vi "find lookahead point - Copy.vi"(6 "Lookahead Distance":dbl=4000.0, 11 "Path Data":T1={"Path"=[], "Target Velocities"=[], "Robot Location"=[], "Robot Angle (rad)"=0.0, "Curvature"=0.0, "Lookahead Point"=[3064.399009129367, 18229.833030071386], "Lookahead Index"=8.422809037111724, "Closest Point"=[], "Closest Point Index"=0, "Left Velocity"=0.0, "Right Velocity"=0.0, "Left Encoder Vel"=0, "Right Encoder Vel"=0, "Left Encoder Pos"=0, "Right Encoder Pos"=0}) -> (3 "Path Data":T1={"Path"=[], "Target Velocities"=[], "Robot Location"=[], "Robot Angle (rad)"=0.0, "Curvature"=0.0, "Lookahead Point"=[3064.399009129367, 18229.833030071386], "Lookahead Index"=8.422809037111724, "Closest Point"=[], "Closest Point Index"=0, "Left Velocity"=0.0, "Right Velocity"=0.0, "Left Encoder Vel"=0, "Right Encoder Vel"=0, "Left Encoder Pos"=0, "Right Encoder Pos"=0})   [LabVIEW 2018]
uses:
  path data.ctl
panel:
  out "a":dbl
  out "Lookahead Index":dbl=8.422809037111724
  out "Lookahead Point":dbl[](array[numeric])=[3064.399009129367, 18229.833030071386]
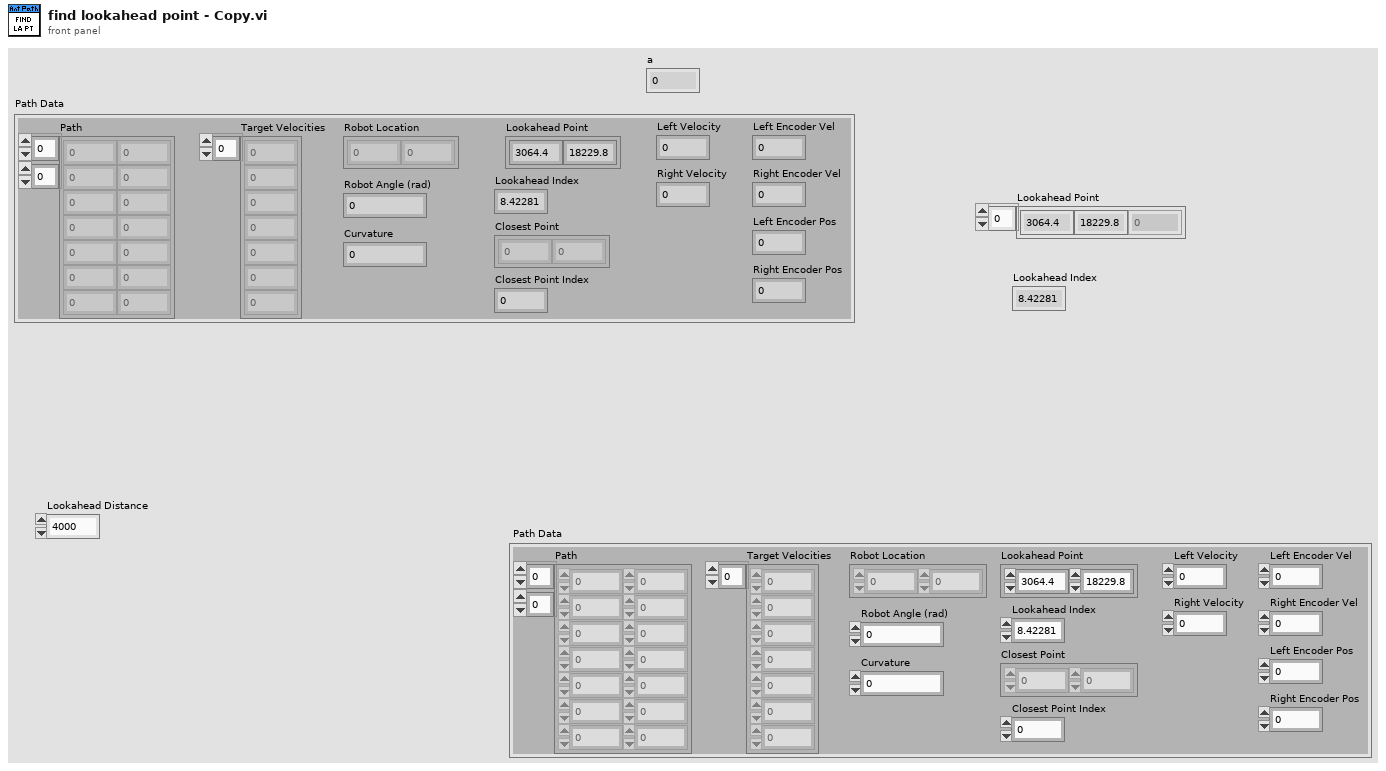
[diagram p1: front panel]
types:
  T1 = typedef "path data.ctl" = cluster{"Path":dbl[][], "Target Velocities":dbl[], "Robot Location":dbl[], "Robot Angle (rad)":dbl, "Curvature":dbl, "Lookahead Point":dbl[], "Lookahead Index":dbl, "Closest Point":dbl[], "Closest Point Index":i32, "Left Velocity":dbl, "Right Velocity":dbl, "Left Encoder Vel":i32, "Right Encoder Vel":i32, "Left Encoder Pos":i32, "Right Encoder Pos":i32}
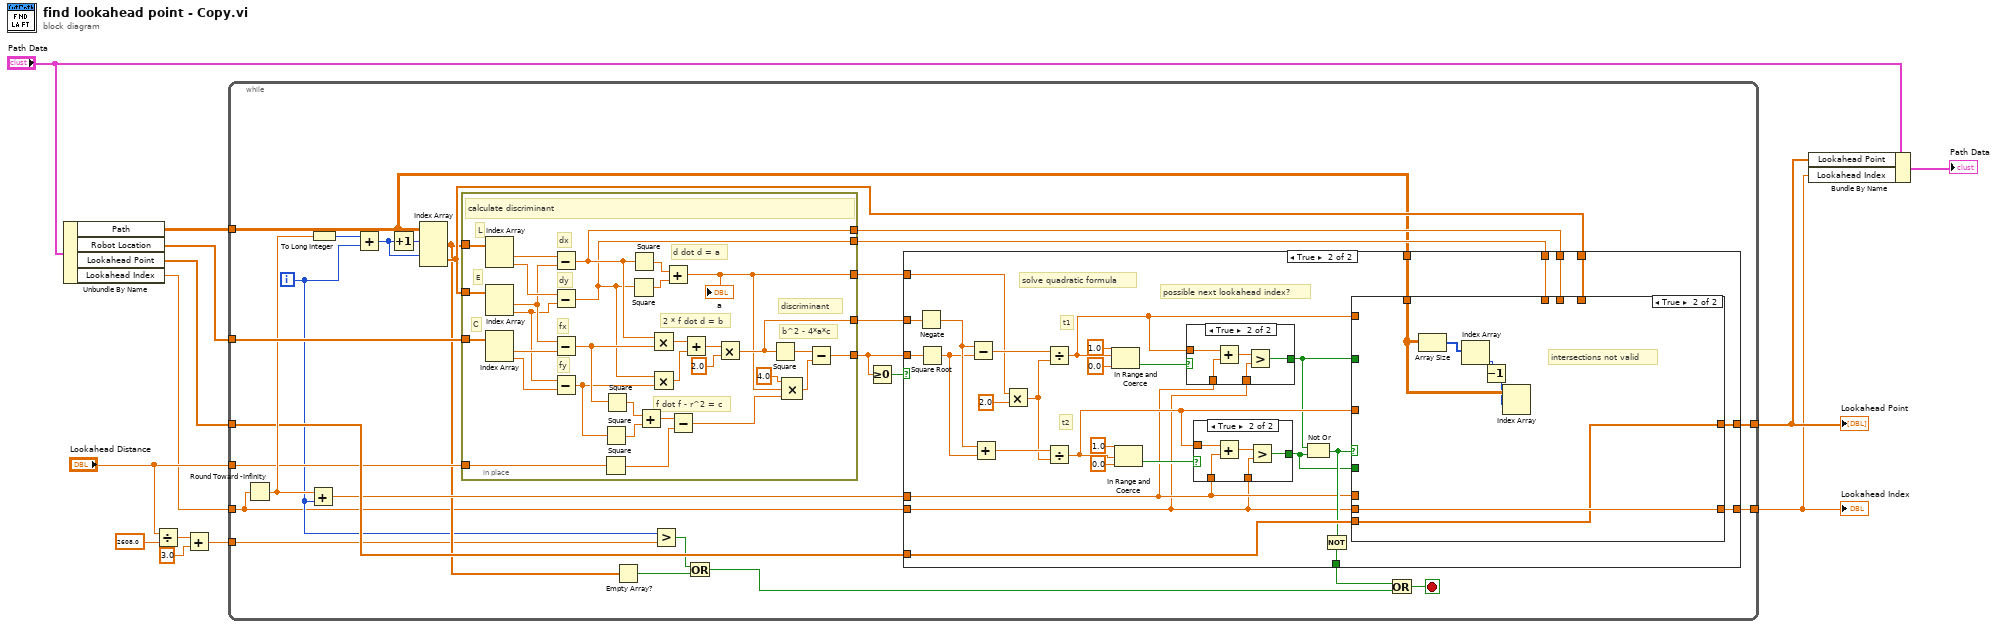
[diagram p0: block diagram]
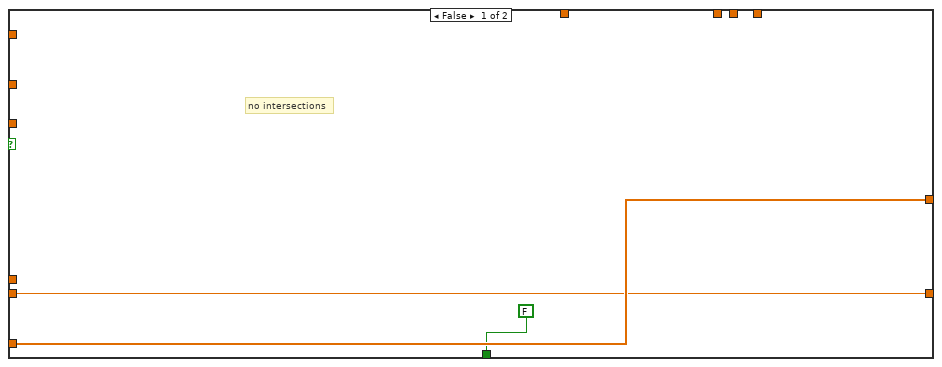
[diagram p2: hidden frame]
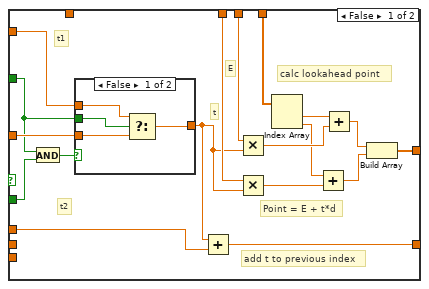
[diagram p3: hidden frame]
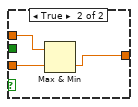
[diagram p4: hidden frame]
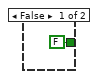
[diagram p5: hidden frame]
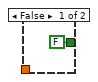
[diagram p6: hidden frame]
diagram:
  n1 = Unbundle By Name("Path Data") -> ("Path"=w4:dbl[][], "Robot Location"=w3:dbl[], "Lookahead Point"=w2:dbl[], "Lookahead Index"=w1:dbl)
  n2 = Divide(x="Lookahead Distance", y=2608.0) -> (x/y=w11:dbl)
  n3 = Add(x=w11, y=3.0) -> (x+y=w9:dbl)
  n4 = while {
    tunnel: w3 -> [w40]
    tunnel: "Lookahead Distance" -> [w30]
    tunnel: w4 -> [w14]
    tunnel: w1 -> [w15]
    tunnel: w2 -> [w33]
    tunnel: [w32] -> w6
    tunnel: [w25] -> w5
    tunnel: w9 -> [w17]
    i -> [w18]
    stop <- w28 stop-if-true
    n5 = Round Toward -Infinity(1:w15) -> (0:w34:dbl)
    n6 = Add(x=w34, y=w18) -> (x+y=w26:dbl)
    n7 = To Long Integer(number=w34) -> (32bit integer=w31:i32)
    n8 = Add(x=w31, y=w18) -> (x+y=w24:i32)
    n9 = Increment(x=w24) -> (x+1=w22:i32)
    n10 = Index Array(array=w14, index (row) #1=w22, index (row) #2=w24) -> (element #1=w21:dbl[], element #2=w23:dbl[])  [unwired: 2 in]
    n11 = in-place {
      in-place-border: w40 -> [w71]
      in-place-border: w30 -> [w54]
      in-place-border: [w47] -> w39
      in-place-border: [w46] -> w38
      in-place-border: [w45] -> w37
      in-place-border: [w44] -> w36
      in-place-border: [w43] -> w35
      in-place-border: w21 -> [w42]
      in-place-border: w23 -> [w41]
      # "C"
      # "E"
      # "L"
      # "calculate discriminant"
      # "b^2 - 4*a*c"
      # "discriminant"
      # "f dot f - r^2 = c"
      # "2 * f dot d = b"
      # "d dot d = a"
      # "fy"
      # "dy"
      # "fx"
      # "dx"
      n12 = Index Array(array=w42) -> (element #1=w70:dbl, element #2=w69:dbl)  [unwired: 2 in]
      n13 = Index Array(array=w41) -> (element #1=w68:dbl, element #2=w66:dbl)  [unwired: 2 in]
      n14 = Index Array(array=w71) -> (element #1=w67:dbl, element #2=w65:dbl)  [unwired: 2 in]
      n15 = Subtract(x=w70, y=w68) -> (x-y=w45:dbl)
      n16 = Subtract(x=w69, y=w66) -> (x-y=w44:dbl)
      n17 = Subtract(x=w68, y=w67) -> (x-y=w58:dbl)
      n18 = Subtract(x=w66, y=w65) -> (x-y=w57:dbl)
      n19 = Square(x=w54) -> (x^2=w53:dbl)
      n20 = Square(x=w57) -> (x^2=w55:dbl)
      n21 = Square(x=w58) -> (x^2=w56:dbl)
      n22 = Square(x=w44) -> (x^2=w64:dbl)
      n23 = Square(x=w45) -> (x^2=w63:dbl)
      n24 = Add(x=w56, y=w55) -> (x+y=w52:dbl)
      n25 = Multiply(x=w45, y=w58) -> (x*y=w62:dbl)
      n26 = Multiply(x=w44, y=w57) -> (x*y=w61:dbl)
      n27 = Add(x=w63, y=w64) -> (x+y=w43:dbl)
      "a" <- w43
      n28 = Subtract(x=w52, y=w53) -> (x-y=w49:dbl)
      n29 = Add(x=w62, y=w61) -> (x+y=w60:dbl)
      n30 = Multiply(x=w60, y=2.0) -> (x*y=w47:dbl)
      n31 = Square(x=w47) -> (x^2=w51:dbl)
      n32 = Compound Arithmetic op=MULTIPLY(4.0 ("value"), w43, w49) -> (w48:dbl)
      n33 = Subtract(x=w51, y=w48) -> (x-y=w46:dbl)
    }
    n34 = Empty Array?(array=w21) -> (empty?=w20:bool)
    n35 = Greater?(x=w18, y=w17) -> (0:w16:bool)
    n36 = Or(x=w16, y=w20) -> (x .or. y?=w19:bool)
    n37 = Greater Or Equal To 0?(x=w38) -> (x >= 0?=w27:bool)
    n38 = case shown="True" w27 {
      tunnel: w33 -> [w74 w90]
      tunnel: [w74 w89] -> w32
      tunnel: w39 -> [_ w98]
      tunnel: w35 -> [_ w85]
      tunnel: w38 -> [_ w97]
      tunnel: w26 -> [_ w77]
      tunnel: w23 -> [_ w88]
      tunnel: w37 -> [_ w87]
      tunnel: w36 -> [_ w86]
      tunnel: w15 -> [w72 w76]
      tunnel: [FALSE w81] -> w29
      tunnel: [w72 w78] -> w25
      tunnel: w14 -> [_ w75]
      frame False {
        # "no intersections"
      }
      frame True {
        # "solve quadratic formula"
        # "possible next lookahead index?"
        # "t2"
        # "t1"
        n39 = Negate(x=w98) -> (-x=w102:dbl)
        n40 = Square Root(x=w97) -> (sqrt(x)=w101:dbl)
        n41 = Subtract(x=w102, y=w101) -> (x-y=w103:dbl)
        n42 = Add(x=w102, y=w101) -> (x+y=w100:dbl)
        n43 = Multiply(x=w85, y=2.0) -> (x*y=w99:dbl)
        n44 = Divide(x=w103, y=w99) -> (x/y=w84:dbl)
        n45 = Divide(x=w100, y=w99) -> (x/y=w83:dbl)
        n46 = In Range and Coerce(upper limit=1.0, x=w84, lower limit=0.0) -> (In Range?=w91:bool)  [unwired: 1 out]
        n47 = In Range and Coerce(upper limit=1.0, x=w83, lower limit=0.0) -> (In Range?=w92:bool)  [unwired: 1 out]
        n48 = case shown="True" w91 {
          tunnel: w84 -> [_ w141]
          tunnel: w77 -> [_ w140]
          tunnel: w76 -> [_ w138]
          tunnel: [FALSE w137] -> w80
          frame False {
          }
          frame True {
            n49 = Add(x=w141, y=w140) -> (x+y=w139:dbl)
            n50 = Greater?(x=w139, y=w138) -> (0:w137:bool)
          }
        }
        n51 = case shown="True" w92 {
          tunnel: w83 -> [_ w147]
          tunnel: w77 -> [_ w146]
          tunnel: w76 -> [_ w144]
          tunnel: [FALSE w143] -> w79
          frame False {
          }
          frame True {
            n52 = Add(x=w147, y=w146) -> (x+y=w145:dbl)
            n53 = Greater?(x=w145, y=w144) -> (0:w143:bool)
          }
        }
        n54 = Not Or(1:w79, 2:w80) -> (0:w82:bool)
        n55 = Not(x=w82) -> (.not. x?=w81:bool)
        n56 = case shown="True" w82 {
          tunnel: w84 -> [w120 _]
          tunnel: w83 -> [w119 _]
          tunnel: w90 -> [_ w130]
          tunnel: [w108 w130] -> w89
          tunnel: w80 -> [w118 _]
          tunnel: w79 -> [w122 _]
          tunnel: w88 -> [w111 _]
          tunnel: w87 -> [w110 _]
          tunnel: w86 -> [w109 _]
          tunnel: [w106 w135] -> w78
          tunnel: w77 -> [w105 _]
          tunnel: w76 -> [_ w135]
          tunnel: w75 -> [_ w134]
          frame False {
            # "add t to previous index"
            # "Point = E + t*d"
            # "calc lookahead point"
            # "t"
            # "t2"
            # "t1"
            # "E"
            n57 = And(x=w118, y=w122) -> (x .and. y?=w121:bool)
            n58 = case shown="False" w121 {
              tunnel: w120 -> [w125 w129]
              tunnel: w119 -> [w124 w128]
              tunnel: [w123 w127] -> w107
              tunnel: w118 -> [w126 _]
              frame False {
                n59 = Select(t=w125, s=w126, f=w124) -> (s? t:f=w123:dbl)
              }
              frame True {
                n60 = Max & Min(x=w129, y=w128) -> (min(x,y)=w127:dbl)  [unwired: 1 out]
              }
            }
            n61 = Add(x=w107, y=w105) -> (x+y=w106:dbl)
            n62 = Multiply(x=w110, y=w107) -> (x*y=w115:dbl)
            n63 = Multiply(x=w109, y=w107) -> (x*y=w114:dbl)
            n64 = Index Array(array=w111) -> (element #1=w113:dbl, element #2=w112:dbl)  [unwired: 2 in]
            n65 = Add(x=w112, y=w114) -> (x+y=w116:dbl)
            n66 = Add(x=w113, y=w115) -> (x+y=w117:dbl)
            n67 = Build Array(w117, w116) -> (w108:dbl[])
          }
          frame True {
            # "intersections not valid"
            n68 = Array Size(array=w134) -> (size(s)=w133:i32[])
            n69 = Index Array(array=w133) -> (element=w132:i32)  [unwired: 1 in]
            n70 = Decrement(x=w132) -> (x-1=w131:i32)
            n71 = Index Array(array=w134, index (row)=w131) -> ()  [unwired: 1 in, 1 out]
          }
        }
      }
    }
    n72 = Or(x=w29, y=w19) -> (x .or. y?=w28:bool)
  }
  "Lookahead Point" <- w6
  "Lookahead Index" <- w5
  n73 = Bundle By Name(cluster="Path Data", "Lookahead Point"=w6, "Lookahead Index"=w5) -> (→"Path Data":T1)
